vi "Retrieve Profiles.vi"   [LabVIEW 2019]
uses:
  Pathfinder-Lib/Pathfinder.lvlib
  Pathfinder-Lib/VIs/Waypoint.ctl
types:
  T1 = typedef "Pathfinder.lvlib/Waypoint.ctl" = cluster{"x":dbl, "y":dbl, "angle":dbl}
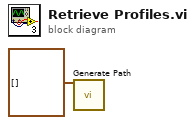
[diagram p0: block diagram]
diagram:
  n1 = call "Generate Path.vi"("path"=T1[] []) -> ()  [unwired: 13 in, 2 out]
